vi "Read Process Variable.vi"(8 "error in (no error)":errorcluster, 10 "Process Variable":u32, 11 "Temp Chamber in":refnum<class "Temp Chamber.lvclass">) -> (0 "error out":errorcluster, 2 "Value":dbl, 3 "Temp Chamber out":refnum<class "Temp Chamber.lvclass">)   [LabVIEW 2018, in "Temp Chamber.lvlib" / "Temp Chamber.lvclass"]
doc: "This Override is used to read a Process Variable value."
uses:
  Temp Chamber.lvclass
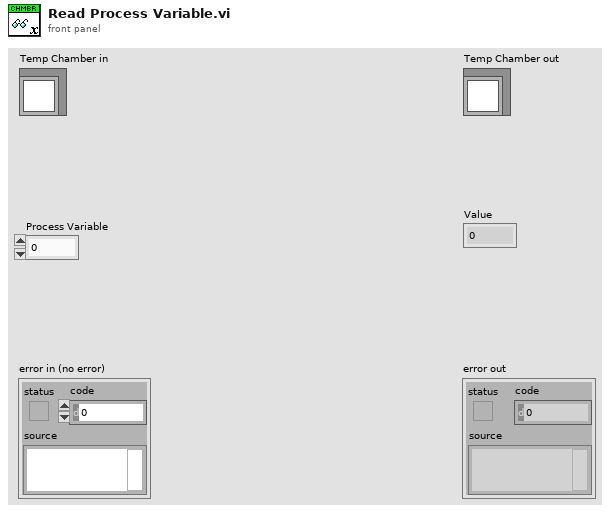
[diagram p1: front panel]
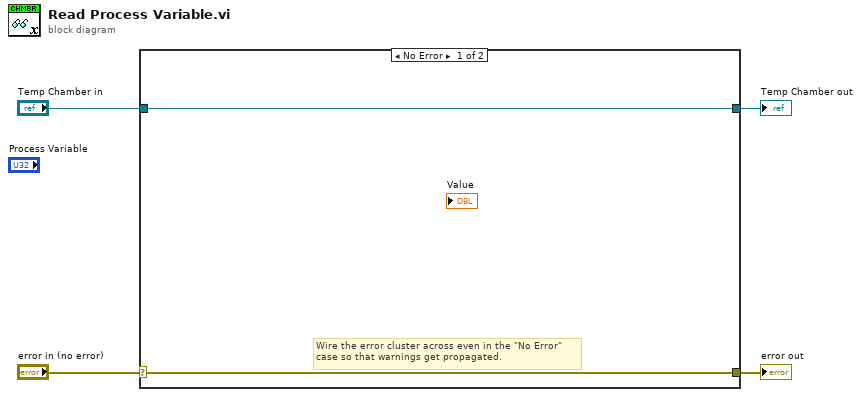
[diagram p0: block diagram]
diagram:
  n1 = case shown="No Error" "error in (no error)" {
    selector: "error in (no error)" -> [w5 w8]
    tunnel: [w5 w8] -> w3
    tunnel: [w6 w7] -> w1
    tunnel: "Temp Chamber in" -> [w6 w7]
    frame No Error {
      # "Wire the error cluster across even in the \"No Error\"\ncase so that warnings get propagated."
    }
    frame Error {
    }
  }
  "error out" <- w3
  "Temp Chamber out" <- w1
